vi "Set UUT Test Evaluation.vi"(8 "error in (no error)":errorcluster, 9 "Pull Passed":bool, 10 "Push Passed":bool, 11 "reference in":refnum<class "UUT.lvclass">) -> (0 "error out":errorcluster, 3 "reference out":refnum<class "UUT.lvclass">)   [LabVIEW 2017, in "UUT.lvclass"]
uses:
  UUT.lvclass
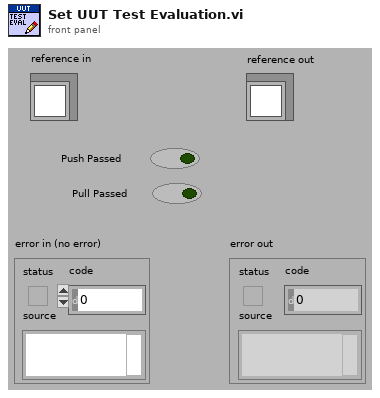
[diagram p1: front panel]
types:
  T1 = typedef "UUT.lvclass/ObjectAttributes.ctl" = cluster{"UUT Info":cluster{"Part Number":string, "Lower Push Limit (lb)":dbl, "Upper Push Limit (lb)":dbl, "Lower Pull Limit (lb)":dbl, "Upper Pull Limit (lb)":dbl, "Push Position (mm)":dbl, "Pull Position (mm)":dbl}, "Test Results":cluster{"Test Time":timestamp, "Number of Trials":u32, "Push Values (lb)":dbl[], "Push Average (lb)":dbl, "Push Std Dev (lb)":dbl, "Push Passed":bool, "Pull Values (lb)":dbl[], "Pull Average (lb)":dbl, "Pull Std Dev (lb)":dbl, "Pull Passed":bool}}
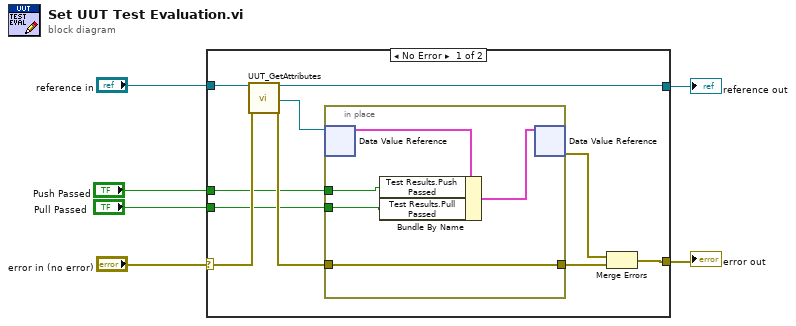
[diagram p0: block diagram]
diagram:
  n1 = case shown="No Error" "error in (no error)" {
    selector: "error in (no error)" -> [w15 w23]
    tunnel: [w12 w23] -> w5
    tunnel: [w13 w22] -> w3
    tunnel: "reference in" -> [w16 w22]
    tunnel: "Push Passed" -> [w8 _]
    tunnel: "Pull Passed" -> [w7 _]
    frame No Error {
      n2 = call "UUT_GetAttributes.vi"("reference in"=w16, "error in (no error)"=w15) -> ("reference out"=w13:refnum<class "UUT.lvclass">, "DataRef"=w11:refnum<data-value>, "error out"=w10:errorcluster)  [unwired: 14 in, 1 out]
      n3 = in-place {
        in-place-border: w10 -> [w21]
        in-place-border: [w21] -> w9
        in-place-border: w8 -> [w18]
        in-place-border: w7 -> [w17]
        n4 = in-place-dvr #1(w11) -> (w20:T1)  [unwired: 1 out]
        n5 = Bundle By Name(cluster=w20, "Test Results.Push Passed"=w18, "Test Results.Pull Passed"=w17) -> (w19:T1)
        n6 = in-place-dvr #1(w19) -> (w14:errorcluster)  [unwired: 1 out]
      }
      n7 = Merge Errors(w14, w9) -> (w12:errorcluster)
    }
    frame Error {
    }
  }
  "error out" <- w5
  "reference out" <- w3
